vi "Get Resolution.vi"(0 "comm interface in":refnum<class "Pixy Com.lvclass">, 11 "error in":errorcluster) -> (4 "comm interface out":refnum<class "Pixy Com.lvclass">, 6 "resolution":cluster{"width":u16, "height":u16}, 15 "error out":errorcluster)   [LabVIEW 2018, in "Pixy2.lvlib"]
uses:
  Pixy2.lvlib
  Interface/Pixy Com.lvclass
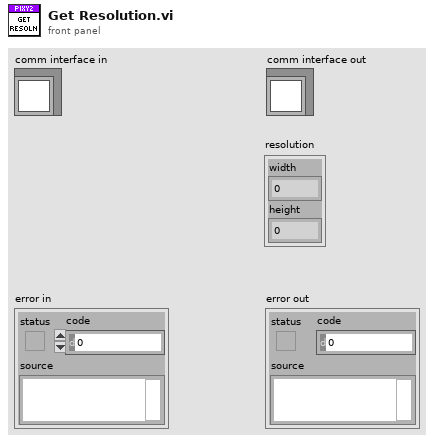
[diagram p1: front panel]
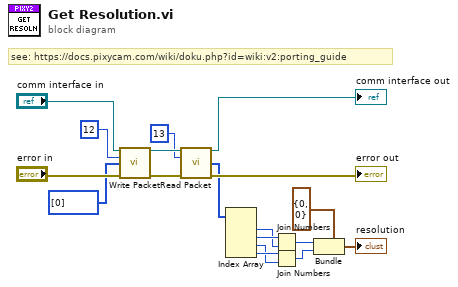
[diagram p0: block diagram]
diagram:
  # "see: https://docs.pixycam.com/wiki/doku.php?id=wiki:v2:porting_guide"
  n1 = call "Write Packet.vi"("comm interface in"="comm interface in", "type"=u8 12, "payload"=u8[] [0], "error in"="error in") -> ("comm interface out"=w15:refnum<class "Pixy Com.lvclass">, "error out"=w16:errorcluster)  [unwired: 10 in]
  n2 = call "Read Packet.vi"("comm interface in"=w15, "expected type"=u8 13, "error in"=w16) -> ("comm interface out"=→"comm interface out":refnum<class "Pixy Com.lvclass">, "received"=w9:u8[], "error out"=→"error out":errorcluster)  [unwired: 9 in, 1 out]
  n3 = Index Array(array=w9) -> (element #1=w7:u8, element #2=w8:u8, element #3=w5:u8, element #4=w6:u8)  [unwired: 4 in]
  n4 = Join Numbers(hi=w8, lo=w7) -> ((hi.lo)=w3:u16)
  n5 = Join Numbers(hi=w6, lo=w5) -> ((hi.lo)=w2:u16)
  n6 = Bundle(cluster=cluster{"width":u16, "height":u16} {"width"=0, "height"=0} ("resolution"), "width"=w3, "height"=w2) -> (→"resolution":cluster{"width":u16, "height":u16})
